vi "ActiView806-Lores.vi"() -> ()   [LabVIEW 2020]
doc: "ActiView is based on a state machine (case structure inside while-loop) with six (orange) states:\n\nState 0: Wait for START, and read/write CFG files\nState 1: Start acquisition, determine speedmode and AD-box version, set panel controls accordingly, stop acquisition\nState 2: Reset panel indicators\nState 3: Initialize saving to BDF file\nState 4: Start acquisition, iterate while-loop to write data to screen and BDF flle (if selected) until STOP is pressed, or error occurs, stop acquisition\nState 5: Reset panel indicators, close BDF file\n\nThe while-loop in (orange) state 4 has five (green) cases.\n\nCase 0: Wait for new data\nCase 1: Read new data from ringbuffer, downsample data, write data to charts and in file array\nCase 2: Transfer block of 1 second of data from file array to BDF file\nCase 3: Close BDF file, and open new BDF file\nCase 4: Calculate average result, and write to ERP graphs \n\nAlso see the Light version of ActiView avalable from the www.biosemi.com"
uses:
  <vilib>/Utility/error.llb/DialogType.ctl
  <vilib>/Utility/config.llb/Read Key (String).vi
  <vilib>/Utility/config.llb/Write Key (String).vi
  <vilib>/Utility/cursorutil.llb/Set Cursor (Icon Pict).vi
  ActiView8-Subvi.llb/StopJazzIni.glb
  ActiView8-Subvi.llb/JazzLoBatWarning.glb
  ActiView8-Subvi.llb/LoBatWarning.glb
  ActiView8-Subvi.llb/StopThreads.glb
  ActiView8-Subvi.llb/TCPidentification.glb
  <vilib>/Utility/inputDevices.llb/keyboardAcquire.vi
  <vilib>/Utility/inputDevices.llb/closeKeyboard.vi
  Instance          61 25Saved   ActiView606-Lores .vi
  <vilib>/Utility/config.llb/NI_LVConfig.lvlib
panel:
  in  "TrigCode":i8(ring) caption="Trigger Format" items=["Analog", "Decimal", "Hexa", "Binary", "Custom"]
  out "Trigger Bar":enum32{"Blank"}(tab)
  out "Dummy String":string
  out "Trigger Chart":i32[][](graph)
  out "Trigger Code":picture
  out "Errors:":i16
  in  "Box":i32(ring) items=["AD-Box 1", "AD-Box 2", "AD-Box 3", "AD-Box 4"]
  out "Right Sidebar":enum32{"Blank"}(tab)
  out "Write":bool
  out "Free on Disk sec":i64=-1 caption="Free on Disc sec"
  out "Nr of Files":i32
  out "Total Saved sec":i32
  out "Current File MB":dbl format="%.1f"
  out "with Jazz":bool
  out "Box4":bool caption="Box1"
  out "Box3":bool caption="Box1"
  out "Box2":bool caption="Box1"
  out "Box1":bool
  in  "FileAppend":bool=TRUE
  in  "RecTimeLimit":i32=9999999 caption="Time Limit (sec)" min=1 max=9999999 step=1
  out "Nr Chan Saved":string="0 + 0"
  out "with AIB":bool
  out "with Sens":bool
  out "with  8 EX":bool
  out "Bandwidth (3dB)":dbl
  in  "Decimation":i8(ring) items=["1", "1/2", "1/4", "1/8", "1/16", "1/32", "1/64"]
  out "Sample Rate":dbl
  in  "FileLimit":i64=999999 caption="File Limit (MB)" min=1 max=999999 step=1
  out "Filepath":string
  out "Save Subset":string
  out "Battery":u8(slide) scale=0.0..100.0
  in  "Marker F8":bool
  in  "Marker F7":bool
  in  "Marker F6":bool
  in  "Marker F5":bool
  in  "Marker F4":bool
  in  "Marker F3":bool
  in  "Marker F2":bool
  in  "Marker F1":bool
  in  "Master Filter Reset":bool
  in  "ScreenLength":i32(ring)=3 caption="Screen Length" items=["1 sec", "2 sec", "4 sec", "8 sec", "16 sec", "32 sec", "64 sec"]
  in  "Start Saving":bool
  in  "Pause Saving":bool
  out "Left Sidebar":T1(tab)
  in  "MonFree":i32[](listbox)=[0, 1, 2, 3, 4, 5, 6, 7, 8, 9, 10, 11, 12, 13, 14, 15, 16, 17, 18, 19, 20, 21, 22, 23, 24, 25, 26, 27, 28, 29, 30, 31, 32, 33, 34, 35, 36, 37, 38, 39, 40, 41, 42, 43, 44, 45, 46, 47, 48, 49, 50, 51, 52, 53, 54, 55, 56, 57, 58, 59, 60, 61, 62, 63, 64, 65, 66, 67, 68, 69, 70, 71, 72, 73, 74, 75, 76, 77, 78, 79, 80, 81, 82, 83, 84, 85, 86, 87, 88, 89, 90, 91, 92, 93, 94, 95, 96, 97, 98, 99, 100, 101, 102, 103, 104, 105, 106, 107, 108, 109, 110, 111, 112, 113, 114, 115, 116, 117, 118, 119, 120, 121, 122, 123, 124, 125, 126, 127, 128, 129, 130, 131, 132, 133, 134, 135, 136, 137, 138, 139, 140, 141, 142, 143, 144, 145, 146, 147, 148, 149, 150, 151, 152, 153, 154, 155, 156, 157, 158, 159, 160, 161, 162, 163, 164, 165, 166, 167, 168, 169, 170, 171, 172, 173, 174, 175, 176, 177, 178, 179, 180, 181, 182, 183, 184, 185, 186, 187, 188, 189, 190, 191, 192, 193, 194, 195, 196, 197, 198, 199, 200, 201, 202, 203, 204, 205, 206, 207, 208, 209, 210, 211, 212, 213, 214, 215, 216, 217, 218, 219, 220, 221, 222, 223, 224, 225, 226, 227, 228, 229, 230, 231, 232, 233, 234, 235, 236, 237, 238, 239, 240, 241, 242, 243, 244, 245, 246, 247, 248, 249, 250, 251, 252, 253, 254, 255]
  in  "Reference":i8(ring) items=["None (raw)", "Avg of 264", "Avg 1-256", "Avg 1-160", "Avg 1-128", "Avg 1-64", "Avg 1-32", "Avg of Displ", "Free Choice"]
  in  "Mon Filter Reset":bool
  in  "MonLP":bool=TRUE caption="Lowpass"
  in  "MonHP":bool=TRUE caption="Highpass"
  in  "RefFree":i32[](listbox)
  in  "Channels":i8(ring) items=["All 264 Chan ", "A-H (256)", "A-E (160)", "ABCD (128)", "A+B (64)", "A (32)", "B (32)", "C (32)", "D (32)", "E (32)", "F (32)", "G (32)", "H(32)", "EXG (8)", "Free Choice"]
  in  "MonHPfreq":dbl=0.16 caption="Cutoff Freq" min=0.01 max=9.99 step=0.1 format="%.2f"
  in  "MonScale":i8(ring)=4 caption="Y-scale\nVolts/div" items=["5 uV", "10 uV", "20 uV", "50 uV", "100 uV", "200 uV", "500 uV", "1 mV", "2 mV", "5 mV", "10 mV", "20 mV", "50 mV", "100 mV", "200 mV", "500 mV"]
  in  "MonLPfreq":dbl=100.0 caption="Cutoff Freq" min=1.0 max=8191.0 step=10.0
  out "NoRef Blinker":bool
  in  "AddTP":bool caption="Add  8 EXG"
  in  "BipFree":i32[](listbox)=[0, 2, 4, 6] caption="Bipolar\nLeads"
  in  "Bip Filter Reset":bool
  in  "BipLP":bool=TRUE caption="Lowpass"
  in  "BipHP":bool=TRUE caption="Highpass"
  in  "BipHPfreq":dbl=0.16 caption="Cutoff Freq" min=0.01 max=99.9 step=1.0 format="%.2f"
  in  "BipScale":i8(ring)=7 caption="Y-scale\nVolts/div" items=["5 uV", "10 uV", "20 uV", "50 uV", "100 uV", "200 uV", "500 uV", "1 mV", "2 mV", "5 mV", "10 mV", "20 mV", "50 mV", "100 mV", "200 mV", "500 mV"]
  in  "BipLPfreq":dbl=100.0 caption="Cutoff Freq" min=1.0 max=8191.0 step=10.0
  out "TP Offset Graph 2":dbl[](graph) caption="EX5 - EX8"
  out "TP Offset Graph 1":dbl[](graph) caption="EX1 - EX4"
  in  "Offset":i8(ring) caption="Channel\nSelection" items=["All 256 Chan ", "A + B", "C + D", "E + F", "G + H"]
  out "Full Range":bool=TRUE
  in  "OffsetScale":i8(ring)=3 caption="Displayed \nRange" items=["20 mV", "50 mV", "100 mV", "262  mV", "1049 mV"]
  out "Rejected Sweeps":i32
  out "Valid Sweeps":i32
  in  "AvgLP":bool caption="Lowpass"
  in  "AvgLPfreq":dbl=100.0 caption="Cuttoff Freq" min=1.0 max=8191.0 step=10.0
  in  "AvgTrigLog":i8(ring) items=["AND trigs ", "OR trigs"]
  in  "AvgTrigSel":i32[](listbox)=[0]
  in  "AvgHP":bool=TRUE caption="Highpass"
  in  "AvgHPfreq":dbl=1.0 caption="Cutoff Freq" min=0.1 max=99.9 step=10.0 format="%.1f"
  out "RejDif":bool caption="Reject"
  out "RejAbs":bool caption="Reject"
  in  "AvgRelReject":dbl=50.0 caption="Difference with\navg more than:" min=0.0 step=1.0 format="%.1f"
  in  "AvgAbsReject":dbl=200.0 caption="All  sweeps\nlarger than:" min=0.0 step=10.0
  in  "AvgSweep":i32=500 caption="Sweep Length" min=1 max=9999 step=100
  in  "AvgAutoscale":bool=TRUE caption="Autoscale"
  in  "AvgScale":dbl=5.0 caption="Y-scale in uV" min=0.0 format="%.1f"
  in  "Averaging":bool
  out "Battery\nCapacitance":u8(slide) caption="Battery" scale=0.0..100.0
  in  "Aux DC Reset":bool
  in  "AuxReset":bool=TRUE caption="Reset at \nScreen Start"
  out "GSR units":string="?"
  out "GSR2":dbl format="%_3f"
  out "GSR1":dbl format="%_3f"
  out "GSR2 pos":bool
  out "GSR2 neg":bool
  out "GSR1 pos":bool
  in  "GsrScale":i8(ring)=4 caption="GSR Y-scale" items=["1", "2", "5", "10", "20", "50", "100", "200", "500", "1k", "2k", "5k", "10k", "20k", "50k", "100k", "200k", "500k", "1M"]
  out "GSR1 neg":bool
  in  "ErgoLP":bool caption="Lowpass"
  in  "ErgoScale":i8(ring)=6 caption="Ergo Y-Scale" items=["5 uV", "10 uV", "20 uV", "50 uV", "100 uV", "200 uV", "500 uV", "1 mV", "2 mV", "5 mV", "10 mV", "20 mV", "50 mV", "100 mV", "200 mV", "500 mV", "1V", "2V", "4V"]
  in  "AuxFree":i32[](listbox)=[0, 1, 2, 3, 4, 5, 6] caption="Sensors"
  out "Degrees Celcius":dbl format="%.2f"
  in  "TempScale":i8(ring)=3 caption="Temp Y-scale" items=["0.01 C", "0.02 C", "0.05  C", "0.1 C", "0.2 C", "0.5 C", "1 C", "2 C", "5  C", "10 C"]
  in  "PletScale":i8(ring)=7 caption="Plet Y-scale" items=["5 uV", "10 uV", "20 uV", "50 uV", "100 uV", "200 uV", "500 uV", "1 mV", "2 mV", "5 mV", "10 mV", "20 mV", "50 mV", "100 mV", "200 mV", "500 mV"]
  in  "RespScale":i8(ring)=4 caption="Resp Y-scale" items=["0.1 mV", "0.2 mV", "0.5  mV", "1 mV", "2 mV", "5 mV", "10 mV", "20 mV", "50 mV", "100 mV", "200 mV", "500 mV"]
  in  "JazzOn":bool caption="Enable Jazz"
  in  "JazzReset":bool=TRUE caption="DC Reset at\nScreen Start"
  in  "Jazz Filter Reset":bool
  in  "JazzFree":i32[](listbox)=[0, 1, 2, 3, 4, 5, 6, 7] caption="Jazz\nChannels"
  out "Jazz Batt Perc":string
  out "Jazz Batt Cap":u8(slide) caption="Jazz Batt" scale=0.0..100.0
  out "Jazz New\nFirmware":bool
  in  "AnaFree":i32[](listbox)=[0, 1, 2, 3, 4, 5, 6, 7, 8, 9, 10, 11, 12, 13, 14, 15] caption="AIB\nChannels"
  in  "AnaReset":bool=TRUE caption="Reset at \nScreen Start"
  out "Ana Offset Graph":dbl[](graph)
  in  "AnaOffset":i32(ring) caption="AIB Channel" items=["Ana1", "Ana2", "Ana3", "Ana4", "Ana5", "Ana6", "Ana7", "Ana8", "Ana9", "Ana10", "Ana11", "Ana12", "Ana13", "Ana14", "Ana15", "Ana16", "Ana17", "Ana18", "Ana19", "Ana20", "Ana21", "Ana22", "Ana23", "Ana24", "Ana25", "Ana26", "Ana27", "Ana28", "Ana29", "Ana30", "Ana31", "Ana32"]
  in  "Ana Filter Reset":bool
  in  "AnaLP":bool=TRUE caption="Lowpass"
  in  "AnaHP":bool=TRUE caption="Highpass"
  in  "AnaHPfreq":dbl=0.16 caption="Cutoff Freq" min=0.01 max=4095.0 step=1.0 format="%.2f"
  in  "AnaScale":i8(ring)=7 caption="Y-scale\nVolts/div" items=["5 uV", "10 uV", "20 uV", "50 uV", "100 uV", "200 uV", "500 uV", "1 mV", "2 mV", "5 mV", "10 mV", "20 mV", "50 mV", "100 mV", "200 mV", "500 mV", "1 V", "2 V", "4 V"]
  in  "AnaLPfreq":dbl=100.0 caption="Cutoff Freq" min=1.0 max=8191.0 step=10.0
  in  "Buffer":i8(ring)=2 caption="Ringbuffer Size" items=["8 Mbyte", "16 Mbyte", "32 Mbyte", "64 Mbyte"]
  out "Pause Off/On":string="-1 / -1"
  out "Write CFG":bool
  in  "Save Configuration File":bool
  out "Current Filepath":string
  in  "Load Configuration File":bool
  in  "Start":bool
  out "Low Battery":bool
  out "CM in Range":bool
  out "Ring Buffer":cluster{dbl, dbl}(knob)={0.0033134730043177896, 0.0033134730043177896} scale=0.0..32.0
  in  "Stop":bool
  in  "Charts/Graphs":T2(tab)
  out "Mon Chart":dbl[][](graph)
  out "Trace61":string
  out "Trace60":string
  out "Trace59":string
  out "Trace58":string
  out "Trace57":string
  out "Trace56":string
  out "Trace55":string
  out "Trace54":string
  out "Trace53":string
  out "Trace52":string
  out "Trace51":string
  out "Trace50":string
  out "Trace49":string
  out "Trace48":string
  out "Trace47":string
  out "Trace46":string
  out "Trace45":string
  out "Trace44":string
  out "Trace43":string
  out "Trace42":string
  out "Trace41":string
  out "Trace40":string
  out "Trace39":string
  out "Trace38":string
  out "Trace37":string
  out "Trace36":string
  out "Trace35":string
  out "Trace34":string
  out "Trace33":string
  out "Trace32":string
  out "Trace31":string
  out "Trace30":string
  out "Trace29":string
  out "Trace28":string
  out "Trace27":string
  out "Trace26":string
  out "Trace25":string
  out "Trace24":string
  out "Trace23":string
  out "Trace22":string
  out "Trace21":string
  out "Trace20":string
  out "Trace19":string
  out "Trace18":string
  out "Trace17":string
  out "Trace16":string
  out "Trace15":string
  out "Trace14":string
  out "Trace13":string
  out "Trace12":string
  out "Trace10":string
  out "Trace9":string
  out "Trace8":string
  out "Trace7":string
  out "Trace6":string
  out "Trace5":string
  out "Trace4":string
  out "Trace3":string
  out "Trace2":string
  out "Trace1":string
  out "Trace64":string
  out "Trace63":string
  out "Trace62":string
  out "Trace11":string
  out "Bip8":string
  out "Bip7":string
  out "Bip6":string
  out "Bip5":string
  out "Bip4":string
  out "Bip3":string
  out "Bip2":string
  out "Bip1":string
  out "Bip Chart":dbl[][](graph)
  out "Offset33":string
  out "Offset64":string
  out "Offset63":string
  out "Offset62":string
  out "Offset61":string
  out "Offset60":string
  out "Offset59":string
  out "Offset58":string
  out "Offset57":string
  out "Offset56":string
  out "Offset55":string
  out "Offset54":string
  out "Offset53":string
  out "Offset52":string
  out "Offset51":string
  out "Offset50":string
  out "Offset49":string
  out "Offset Graph First Half":dbl[](graph)
  out "Offset48":string
  out "Offset47":string
  out "Offset46":string
  out "Offset45":string
  out "Offset44":string
  out "Offset43":string
  out "Offset42":string
  out "Offset41":string
  out "Offset40":string
  out "Offset39":string
  out "Offset38":string
  out "Offset37":string
  out "Offset36":string
  out "Offset35":string
  out "Offset34":string
  out "Offset32":string
  out "Offset31":string
  out "Offset30":string
  out "Offset29":string
  out "Offset28":string
  out "Offset27":string
  out "Offset26":string
  out "Offset25":string
  out "Offset24":string
  out "Offset23":string
  out "Offset22":string
  out "Offset21":string
  out "Offset20":string
  out "Offset19":string
  out "Offset18":string
  out "Offset17":string
  out "Offset16":string
  out "Offset15":string
  out "Offset14":string
  out "Offset13":string
  out "Offset12":string
  out "Offset11":string
  out "Offset10":string
  out "Offset9":string
  out "Offset8":string
  out "Offset7":string
  out "Offset6":string
  out "Offset5":string
  out "Offset4":string
  out "Offset3":string
  out "Offset2":string
  out "Offset1":string
  out "Offset Graph  Second Half":dbl[](graph)
  out "Avg2":dbl[][](graph) caption="Avg 2"
  out "Avg1":dbl[][](graph) caption="Avg 1"
  in  "RefFreeAvg2":i32[](listbox)
  in  "MonFreeAvg2":i32(listbox)=1
  in  "RefFreeAvg1":i32[](listbox)
  in  "MonFreeAvg1":i32(listbox)
  out "Sweeping":bool
  out "Aux7":string
  out "Aux6":string
  out "Aux5":string
  out "Aux4":string
  out "Aux Chart":dbl[][](graph)
  out "Aux3":string
  out "Aux2":string
  out "Aux1":string
  out "Jazz9":string
  out "Jazz8":string
  out "Jazz7":string
  out "Jazz6":string
  out "Jazz5":string
  out "Jazz4":string
  out "Jazz Chart":dbl[][](graph)
  out "Jazz3":string
  out "Jazz2":string
  out "Jazz1":string
  out "Ana17":string
  out "Ana18":string
  out "Ana19":string
  out "Ana20":string
  out "Ana21":string
  out "Ana32":string
  out "Ana31":string
  out "Ana30":string
  out "Ana29":string
  out "Ana28":string
  out "Ana27":string
  out "Ana26":string
  out "Ana25":string
  out "Ana22":string
  out "Ana23":string
  out "Ana24":string
  out "Ana Chart":dbl[][](graph)
  out "Ana1":string
  out "Ana2":string
  out "Ana3":string
  out "Ana4":string
  out "Ana5":string
  out "Ana16":string
  out "Ana15":string
  out "Ana14":string
  out "Ana13":string
  out "Ana12":string
  out "Ana11":string
  out "Ana10":string
  out "Ana9":string
  out "Ana6":string
  out "Ana7":string
  out "Ana8":string
  in  "TCPaddJazz":bool caption="Add 9 Jazz"
  in  "TCPaddTrig":bool caption="Add Trigger/Status Chan"
  out "Bytes in TCP Array":i32
  out "Bytes received by Client":i32
  out "TCP samples/channel":i32
  out "Channels sent by TCP":i32
  in  "TCPaddAnas":bool caption="Add 32 AIB Chan"
  in  "TCPaddSens":bool caption="Add 7 Sensors"
  in  "TCPaddTP":bool caption="Add  8 EX  electrodes"
  in  "TCPsubset":i8(ring)=7 caption="TCP subset:" items=["A1 - H32 (256)", "A1 - E32 (160)", "A1 - D32 (128)", "A1 - B32 (64)", "A1 - A32 (32)", "A1 - A16 (16)", "A1 -A8 (8)", "None (0) "]
  out "TCP Listening":bool
  out "TCP Connected":bool
  out "Remote Address":string
  out "Receive Remote Port":u16
  out "Bytes sent by Server":i32
  in  "LocalPort":u16=778 caption="Sent Local Port"
  out "Application:Kind":T3(ring)
  out "AD-box":string="?"
  out "Speed Mode":i8=-1
  in  "Edit":bool
  # "Trig 1 - 8"
  # "Trig 9-16"
  # "BDF File"
  # "Hz"
  # "Hz"
  # "AD-Box"
  # "Hz"
  # "Hz"
  # "None = CMS"
  # "Hz"
  # "Hz"
  # "ms"
  # "Hz"
  # "Hz"
  # "uV"
  # "uV"
  # "uV"
  # "GSR\nIn Range"
  # "1"
  # "2"
  # "C"
  # "Hz"
  # "Hz"
  # "Range in mV"
  # "Versus"
  # "Versus"
  # "ActiView"
  # "data-acquisition software for ActiveTwo measurement system"
  # "Version 8.0, February 13, 2018"
  # "Push to edit source code (LabVIEW licensees only)"
  # "www.biosemi.com\nmetting@biosemi.com\n+31 20 3302956\n+31 650 626354 (emergencies)"
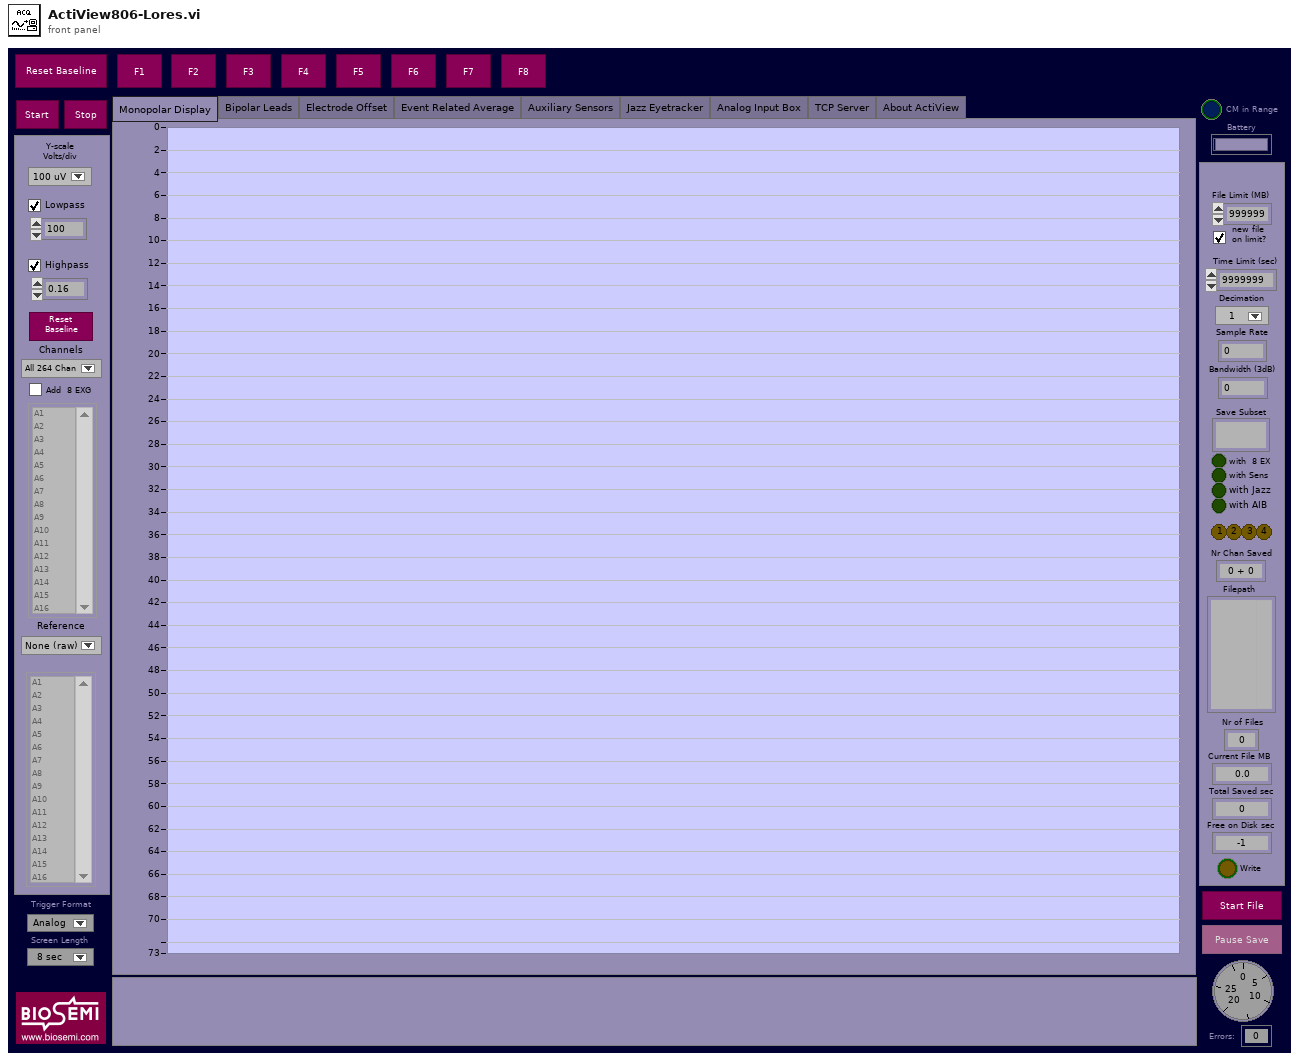
[diagram p1: front panel]
types:
  T1 = enum32{"Monopolar", "Bipolar", "Offset", "Average", "Sensors", "Jazz", "Analog", "Initialization"}
  T2 = enum32{"Monopolar Display", "Bipolar Leads", "Electrode Offset", "Event Related Average", "Auxiliary Sensors", "Jazz Eyetracker", "Analog Input Box", "TCP Server", "About ActiView"}
  T3 = enum32{"invalid app kind", "Development System", "Run Time System", "Student Edition", "Embedded LabVIEW", "Evaluation", "Custom"}
  T4 = enum32{"Page Enabled", "Page Disabled", "Page Disabled & Grayed"}
  T5 = enum8{"Enabled", "Disabled", "Disabled and Grayed Out"}
  T6 = cluster{"Warning":i8, "Motherboard":i8, "ElecGain":i8, "RespSwitch":i8, "LineWidth":u8, "Cursor":u16, "PopupKiller":i8, "BreathBelt":i8}
  T7 = cluster{"Mark2":bool, "GSR16Hz":bool, "JazzRec":bool, "Speed Mode":i8, "ADC Rate":i32, "ADC Channels":i32, "Screen Ratio":i32, "Decimate Ratio":i32, "Mon Channels":i32, "Bip Channels":i32, "Aux Channels":i32, "Jazz Channels":i32, "Ana Channels":i32, "Save Subset":i8, "Add Touchproofs":bool, "Add Sensors":bool, "Add Jazz":bool, "Add Anas":bool, "Save Box":u32, "PauseOff":i32, "PauseOn":i32, "Save Path":path}
  T8 = cluster{"All Labels":string[], "Spec Labels":string[]}
  T9 = cluster{"connection ID":refnum<k5>, "remote address":string, "remote port":u16}
  T10 = enum16{"open", "replace", "create", "open or create", "replace or create", "replace or create with confirmation"}
  T11 = cluster{"Start Averaging":bool, "Busy Averaging":bool, "Sweep Lenght in Samples":i32, "Valid Sweeps":i32, "Rejected Sweeps":i32, "First Graph Update":bool}
  T12 = enum16{"0", "1", "2", "3", "4", "5", "6", "7", "8", "9", "A", "B", "C", "D", "E", "F", "G", "H", "I", "J", "K", "L", "M", "N", "O", "P", "Q", "R", "S", "T", "U", "V", "W", "X", "Y", "Z", "F1", "F2", "F3", "F4", "F5", "F6", "F7", "F8", "F9", "F10", "F11", "F12", "F13", "F14", "F15", "ADD", "BACK", "BACKSLASH", "CAPITAL", "COMMA", "DECIMAL", "DELETE", "DIVIDE", "DOWN", "END", "EQUALS", "ESCAPE", "GRAVE (`)", "HOME", "INSERT", "LBRACKET", "LCONTROL", "LEFT", "L ALT", "LSHIFT", "LWIN", "MINUS", "MULTIPLY", "NEXT", "NUMLOCK", "NUMPAD_0", "NUMPAD_1", "NUMPAD_2", "NUMPAD_3", "NUMPAD_4", "NUMPAD_5", "NUMPAD_6", "NUMPAD_7", "NUMPAD_8", "NUMPAD_9", "PAUSE", "PERIOD", "PRIOR (PG UP)", "RBRACKET", "RCONTROL", "RETURN", "RIGHT", "R ALT", "RSHIFT", "RWIN", "SCROLL", "SEMICOLON", "SLASH", "SPACE", "SUBTRACT", "TAB", "UP", "ENTER (num pad)", "' (quote)"}
  T13 = cluster{"Font Name:":string, "Size":i16, "Strikeout?":bool, "Italic?":bool, "Underline?":bool, "Outline?":bool, "Shadow?":bool, "Bold?":bool}
  T14 = cluster{"Jazz No Data":bool, "Jazz Packet Loss":bool, "Jazz Batt":u8, "Jazz Packet Loss 2":bool}
  T15 = cluster{"GSR2pos":bool, "GSR1neg":bool, "GSR1pos":bool, "GSR2neg":bool}
  T16 = cluster{"Sweeping":bool, "RejAbs":bool, "RejDif":bool}
  T17 = cluster{"Speed Mode":i8, "Save Subset":i8, "Initially Channel Selection":i32[], "Add Touchproofs":bool, "Mon Channels":i32, "Bip Channels":i32, "Add Sensors":bool, "Initially Channel Selection":i32[], "Add Jazz":bool, "Initially Channel Selection":i32[], "Add Anas":bool, "Initially Channel Selection":i32[], "Save Box":u32}
  T18 = typedef "DialogType.ctl" = u16
  T19 = typedef "NI_LVConfig.lvlib/Config Data RefNum.ctl" = refnum<k1>
  T20 = cluster{"Save Subset":i8, "Add Touchproofs":bool, "Add Sensors":bool, "Add Jazz":bool, "Add Anas":bool, "Save Box":u32}
  T21 = cluster{"Local Patient Identification":string, "Local  Recording Identification":string}
  T22 = cluster{"Mark2":bool, "GSR16Hz":bool, bool, "Speed Mode":i8}
  T23 = typedef "AVTCP-TCP Options.ctl" = cluster{"Subset":i32, "EX":bool}
  T24 = cluster{"length":i32, "f":i32, "f":i32, "f":i32, "f":i32, "f":i32}
  T25 = cluster{bool, bool, bool, bool, bool, bool, bool, bool}
  T26 = cluster{"Clear Block":i32, "Screen Ratio":dbl, "Y1":i16, "Y2":i16, "Y3":i16, "Color":u32}
  T27 = cluster{"Sync Errors":i16, "Recent Sync Error":bool}
  T28 = cluster{"LoBatChange":bool, "JazzLoBatChange":bool}
  T29 = enum16{"0", "1", "2", "3", "4", "5", "6", "7", "8", "9", "A", "B", "C", "D", "E", "F", "G", "H", "I", "J", "K", "L", "M", "N", "O", "P", "Q", "R", "S", "T", "U", "V", "W", "X", "Y", "Z", "F1", "F2", "F3", "F4", "F5", "F6", "F7", "F8", "F9", "F10", "F11", "F12", "F13", "F14", "F15", "ADD", "BACK", "BACKSLASH", "CAPITAL", "COMMA", "DECIMAL", "DELETE", "DIVIDE", "DOWN", "END", "EQUALS", "ESCAPE", "GRAVE (`)", "HOME", "INSERT", "LBRACKET", "LCONTROL", "LEFT", "L ALT", "LSHIFT", "LWIN", "MINUS", "MULTIPLY", "NEXT", "NUMLOCK", "NUMPAD_0", "NUMPAD_1", "NUMPAD_2", "NUMPAD_3", "NUMPAD_4", "NUMPAD_5", "NUMPAD_6", "NUMPAD_7", "NUMPAD_8", "NUMPAD_9", "PAUSE", "PERIOD", "PRIOR (PG UP)", "RBRACKET", "RCONTROL", "RETURN", "RIGHT", "R ALT", "RSHIFT", "RWIN", "SCROLL", "SEMICOLON", "SLASH", "SPACE", "SUBTRACT", "TAB", "UP", "ENTER (num pad)", "' (quote)"}[]
  T30 = cluster{"GsrScale":i8, "ErgoScale":i8, "ErgoLP":bool, "RespScale":i8, "PletScale":i8, "TempScale":i8}
  T31 = cluster{"Mon Channels":i32, "Bip Channels":i32, "Aux Channels":i32, "Jazz Channels":i32}
  T32 = cluster{"End of Screen":bool, "Prop Screen Minimum":i64, "Screen Position":i32}
  T33 = cluster{"Ring Buffer Overflow":bool, "First Call":bool}
  T34 = cluster{"GSR1pos":bool, "GSR1neg":bool, "GSR2pos":bool, "GSR2neg":bool}
  T35 = cluster{"Jazz No Data":bool, "Jazz Packet Loss":bool, "Jazz Batt":u8, "Jazz New Firmware":bool}
  T36 = cluster{"Xo":dbl, "Xmax":dbl, "Xmin":dbl, "Marker values":dbl[]}
  T37 = cluster{"AvgLP":bool, "AvgLPfreq ":dbl, "AvgHP":bool, "AvgHPfreq":dbl}
  T38 = cluster{"MonLP":bool, "MonLPfreq":dbl, "MonHP":bool, "MonHPfreq":dbl}
  T39 = cluster{"BipLP":bool, "BipLPfreq":dbl, "BipHP":bool, "BipHPfreq":dbl}
  T40 = cluster{"AnaLP":bool, "AnaLPfreq":dbl, "AnaHP":bool, "AnaHPfreq":dbl}
  T41 = cluster{"Speed Mode":i8, "Save Subset":i8, i32[], "Add Touchproofs":bool, "Mon Channels":i32, "Bip Channels":i32, "Add Sensors":bool, i32[], "Add Jazz":bool, i32[], "Add Anas":bool, i32[], "Save Box":u32}
  T42 = cluster{"Marker F1":bool, "Marker F2":bool, "Marker F3":bool, "Marker F4":bool, "Marker F5":bool, "Marker F6":bool, "Marker F7":bool, "Marker F8":bool}
diagram:
  w2 = i8 0  # BreathBelt
  w4 = FALSE  # JazzRec
  w7 = FALSE  # Add Anas
  w9 = 0  # Ana Channels
  w5 = FALSE  # GSR16Hz
  w14 = u32 0  # Save Box
  w6 = FALSE  # Mark2
  w17 = path ""  # Save Path
  w15 = 0  # PauseOff
  w16 = 0  # PauseOn
  w19 = 0  # ADC Rate
  w20 = 0  # ADC Channels
  w22 = 0  # Screen Ratio
  w8 = FALSE  # Add Jazz
  w10 = 0  # Jazz Channels
  w11 = FALSE  # Add Sensors
  w12 = FALSE  # Add Touchproofs
  w13 = i8 0  # Save Subset
  w18 = i8 -1  # Speed Mode
  w21 = 0  # Aux Channels
  w24 = 0  # Bip Channels
  w23 = 0  # Decimate Ratio
  w25 = 0  # Mon Channels
  w26 = i8 0  # PopupKiller
  w31 = FALSE  # Initially Not Start with Save
  w34 = refnum<file> refnum  # Dummy Refnum
  w27 = u16 0  # Cursor
  w28 = u8 0  # LineWidth
  w29 = i8 -1  # RespSwitch
  w37 = i8 -1  # Warning
  w39 = i8 -1  # Motherboard
  w38 = i8 -1  # ElecGain
  w40 = FALSE  # Initially Not Config Changed
  w42 = string[] []  # Spec Labels
  w43 = string[] []  # All Labels
  w30 = i32[] []  # Initially Channel Selection
  w32 = 0  # Initially  nothing saved
  w45 = FALSE  # Initially Not Busy Saving
  w44 = 0  # Initial State
  n1 = stacked-sequence {
    tunnel: [w74] -> w35
    frame #0 {
      w46 = T5."Enabled" ("Disabled")
      w47 = 0.5 ("X Scale.Range:Minimum")
      w48 = 128.5 ("X Scale.Range:Maximum")
      w51 = 8191.0 ("Data Range:Maximum")
      w74 = errorcluster {"status"=FALSE, "code"=0, "source"=""}  # Initially  No Error
      w75 = i32[] [] ("Disabled Items []")
      w72 = FALSE ("Visible")
      n2 = for {
        N: 264 -> [_]
        tunnel: [w90] -> w76 mode=indexing
        i -> [w95]
        n3 = Quotient & Remainder(x=w95, y=32) -> (x-y*floor(x/y)=w92:i32, floor(x/y)=w93:i32)
        n4 = case shown="8" w93 {
          tunnel: ["A" "B" "C" "D" "E" "F" "G" "H" "EX"] -> w91
          frame 0, Default {
          }
          frame 1 {
          }
          frame 2 {
          }
          frame 3 {
          }
          frame 4 {
          }
          frame 5 {
          }
          frame 6 {
          }
          frame 7 {
          }
          frame 8 {
          }
        }
        n5 = Increment(x=w92) -> (x+1=w89:i32)
        n6 = Format Into String(initial string=w91, w89) -> (resulting string=w90:string)  [unwired: 2 in, 1 out]
      }
      n7 = for {
        N: 128 -> [_]
        tunnel: [w79] -> w49 mode=indexing
        i -> [w81]
        n8 = Increment(x=w81) -> (x+1=w80:i32)
        n9 = To Double Precision Float(number=w80) -> (double precision float=w79:dbl)
      }
      n10 = Increment(x=264) -> (x+1=w56:i32)
      n11 = Increment(x=8) -> (x+1=w55:i32)
      n12 = Increment(x=7) -> (x+1=w54:i32)
      n13 = Increment(x=9) -> (x+1=w53:i32)
      n14 = Increment(x=32) -> (x+1=w52:i32)
      n15 = property on="Charts/Graphs" class="TabCtl (strict)"() -> ("Pages"=w73:refnum<vi>[])  [unwired: 2 in, 2 out]
      n16 = property on="Low Battery" class="Bool (strict)"("Visible"=w72) -> ()  [unwired: 2 in, 2 out]
      n17 = for {
        N: w54 -> [_]
        tunnel: [w84] -> w64 mode=indexing
        i -> [w84]
      }
      n18 = for {
        N: w53 -> [_]
        tunnel: [w83] -> w61 mode=indexing
        i -> [w83]
      }
      n19 = property on="NoRef Blinker" class="Bool"("Visible"=w72) -> ()  [unwired: 2 in, 2 out]
      n20 = property on="Box" class="Ring (strict)"("Visible"=w72) -> ()  [unwired: 2 in, 2 out]
      n21 = for {
        N: w55 -> [_]
        tunnel: [w85] -> w67 mode=indexing
        i -> [w85]
      }
      n22 = for {
        N: w52 -> [_]
        tunnel: [w82] -> w58 mode=indexing
        i -> [w82]
      }
      n23 = for {
        N: w56 -> [_]
        tunnel: [w86] -> w70 mode=indexing
        i -> [w86]
      }
      n24 = for {
        tunnel: w73 -> [w88] mode=indexing
        n25 = property class="Page"(reference=w88, "Page Enabled State"=T4."Page Enabled") -> ()  [unwired: 1 in, 2 out]
      }
      n26 = property on="AddTP" class="Bool (strict)"("Disabled"=w46) -> ()  [unwired: 2 in, 2 out]
      n27 = property on="TP Offset Graph 1" class="WFGraph (strict)"("Disabled"=w46) -> ()  [unwired: 2 in, 2 out]
      n28 = property on="TP Offset Graph 2" class="WFGraph (strict)"("Disabled"=w46) -> ()  [unwired: 2 in, 2 out]
      n29 = property on="GSR1 pos" class="Bool (strict)"("Disabled"=w46) -> ()  [unwired: 2 in, 2 out]
      n30 = property on="GSR1 neg" class="Bool (strict)"("Disabled"=w46) -> ()  [unwired: 2 in, 2 out]
      n31 = property on="GSR1" class="DigNum (strict)"("Disabled"=w46) -> ()  [unwired: 2 in, 2 out]
      n32 = property on="GSR2 neg" class="Bool (strict)"("Disabled"=w46) -> ()  [unwired: 2 in, 2 out]
      n33 = property on="GSR2 pos" class="Bool (strict)"("Disabled"=w46) -> ()  [unwired: 2 in, 2 out]
      n34 = property on="GsrScale" class="Ring (strict)"("Disabled"=w46) -> ()  [unwired: 2 in, 2 out]
      n35 = property on="GSR units" class="Str"("Disabled"=w46) -> ()  [unwired: 2 in, 2 out]
      n36 = property on="ErgoScale" class="Ring (strict)"("Disabled"=w46) -> ()  [unwired: 2 in, 2 out]
      n37 = property on="ErgoLP" class="Bool (strict)"("Disabled"=w46) -> ()  [unwired: 2 in, 2 out]
      n38 = property on="RespScale" class="Ring (strict)"("Disabled"=w46) -> ()  [unwired: 2 in, 2 out]
      n39 = property on="PletScale" class="Ring (strict)"("Disabled"=w46) -> ()  [unwired: 2 in, 2 out]
      n40 = property on="TempScale" class="Ring (strict)"("Disabled"=w46) -> ()  [unwired: 2 in, 2 out]
      n41 = property on="Degrees Celcius" class="DigNum (strict)"("Disabled"=w46) -> ()  [unwired: 2 in, 2 out]
      n42 = property on="JazzOn" class="Bool (strict)"("Disabled"=w46) -> ()  [unwired: 2 in, 2 out]
      n43 = To Double Precision Float(number=w70) -> (double precision float=w69:dbl[])
      n44 = To Double Precision Float(number=w67) -> (double precision float=w66:dbl[])
      n45 = To Double Precision Float(number=w64) -> (double precision float=w63:dbl[])
      n46 = To Double Precision Float(number=w61) -> (double precision float=w60:dbl[])
      n47 = To Double Precision Float(number=w58) -> (double precision float=w57:dbl[])
      n48 = property on="ScreenLength" class="Ring (strict)"("Disabled Items []"=w75) -> ()  [unwired: 2 in, 2 out]
      n49 = property on="Channels" class="Ring (strict)"("Disabled Items []"=w75) -> ()  [unwired: 2 in, 2 out]
      n50 = property on="Reference" class="Ring (strict)"("Disabled Items []"=w75) -> ()  [unwired: 2 in, 2 out]
      n51 = property on="Offset" class="Ring (strict)"("Disabled Items []"=w75) -> ()  [unwired: 2 in, 2 out]
      n52 = property on="TCPsubset" class="Ring (strict)"("Disabled Items []"=w75) -> ()  [unwired: 2 in, 2 out]
      n53 = property on="Offset Graph First Half" class="WFGraph (strict)"("XScale.Maximum"=w48, "XScale.Minimum"=w47, "XScale.MarkerVals[]"=w49) -> ()  [unwired: 2 in, 2 out]
      n54 = property on="Offset Graph  Second Half" class="WFGraph (strict)"("XScale.Maximum"=w48, "XScale.Minimum"=w47, "XScale.MarkerVals[]"=w49) -> ()  [unwired: 2 in, 2 out]
      n55 = property on="Mon Chart" class="WFChart (strict)"("YScale.MarkerVals[]"=w69) -> ()  [unwired: 2 in, 2 out]
      n56 = property on="Bip Chart" class="WFChart (strict)"("YScale.MarkerVals[]"=w66) -> ()  [unwired: 2 in, 2 out]
      n57 = property on="Aux Chart" class="WFChart (strict)"("YScale.MarkerVals[]"=w63) -> ()  [unwired: 2 in, 2 out]
      n58 = property on="Jazz Chart" class="WFChart (strict)"("YScale.MarkerVals[]"=w60) -> ()  [unwired: 2 in, 2 out]
      n59 = property on="Ana Chart" class="WFChart (strict)"("YScale.MarkerVals[]"=w57) -> ()  [unwired: 2 in, 2 out]
      n60 = property on="BipLPfreq" class="DigNum (strict)"("Data Range:Maximum"=w51) -> ()  [unwired: 2 in, 2 out]
      n61 = property on="AvgLPfreq" class="DigNum (strict)"("Data Range:Maximum"=w51) -> ()  [unwired: 2 in, 2 out]
      n62 = property on="AnaLPfreq" class="DigNum (strict)"("Data Range:Maximum"=w51) -> ()  [unwired: 2 in, 2 out]
      n63 = property on="MonLPfreq" class="DigNum (strict)"("Data Range:Maximum"=w51) -> ()  [unwired: 2 in, 2 out]
      n64 = property on="MonFree" class="LstBox (strict)"("Item Names"=w76) -> ()  [unwired: 2 in, 2 out]
      n65 = property on="RefFree" class="LstBox (strict)"("Item Names"=w76) -> ()  [unwired: 2 in, 2 out]
      n66 = property on="MonFreeAvg1" class="LstBox (strict)"("Item Names"=w76) -> ()  [unwired: 2 in, 2 out]
      n67 = property on="RefFreeAvg1" class="LstBox (strict)"("Item Names"=w76) -> ()  [unwired: 2 in, 2 out]
      n68 = property on="MonFreeAvg2" class="LstBox (strict)"("Item Names"=w76) -> ()  [unwired: 2 in, 2 out]
      n69 = property on="RefFreeAvg2" class="LstBox (strict)"("Item Names"=w76) -> ()  [unwired: 2 in, 2 out]
      n70 = property on="Battery" class="Slide (strict)"("Visible"=TRUE) -> ()  [unwired: 2 in, 2 out]
    }
  }
  n71 = vi-ref "AVTCP-Server.vi"() -> (w1:refnum<vi>)
  n72 = invoke on="Control server" class="SubPnl" method="Insert VI"("VI Ref"=w1) -> ()  [unwired: 3 in, 4 out]
  n73 = call "AVTCP-Server.vi"() -> ()  [unwired: 12 in]
  n74 = Bundle("Warning"=w37, "Motherboard"=w39, "ElecGain"=w38, "RespSwitch"=w29, "LineWidth"=w28, "Cursor"=w27, "PopupKiller"=w26, "BreathBelt"=w2) -> (w36:T6)  [unwired: 1 out]
  n75 = Bundle("Mark2"=w6, "GSR16Hz"=w5, "JazzRec"=w4, "Speed Mode"=w18, "ADC Rate"=w19, "ADC Channels"=w20, "Screen Ratio"=w22, "Decimate Ratio"=w23, "Mon Channels"=w25, "Bip Channels"=w24, "Aux Channels"=w21, "Jazz Channels"=w10, "Ana Channels"=w9, "Save Subset"=w13, "Add Touchproofs"=w12, "Add Sensors"=w11, "Add Jazz"=w8, "Add Anas"=w7, "Save Box"=w14, "PauseOff"=w15, "PauseOn"=w16, "Save Path"=w17) -> (w3:T7)  [unwired: 1 out]
  n76 = Bundle("All Labels"=w43, "Spec Labels"=w42) -> (w41:T8)  [unwired: 1 out]
  n77 = To Quad Integer(1:w32) -> (0:w33:i64)
  n78 = while {
    shift-left: w32 -> [w144]
    shift-right: [w143] -> _
    shift-left: w33 -> [w148]
    shift-right: [w149] -> _
    shift-left: w41 -> [w154]
    shift-right: [w155] -> _
    shift-left: w3 -> [w125]
    shift-right: [w156] -> _
    shift-left: w35 -> [w146]
    shift-right: [w157] -> _
    shift-left: w34 -> [w159]
    shift-right: [w158] -> _
    shift-left: w45 -> [w161]
    shift-right: [w160] -> _
    shift-left: w44 -> [w163]
    shift-right: [w162] -> _
    shift-right: [w140] -> _
    shift-left: w30 -> [w122]
    shift-right: [w135] -> _
    shift-left: w30 -> [w119]
    shift-right: [w133] -> _
    shift-left: w40 -> [w134]
    shift-right: [w132] -> _
    shift-left: w30 -> [w117]
    shift-right: [w127] -> _
    shift-left: w36 -> [w128]
    shift-right: [w115] -> _
    shift-left: w31 -> [w114]
    shift-right: [w113] -> _
    shift-left: w30 -> [w106]
    stop <- w147 stop-if-true
    w126 = 3  # Bytes per Word
    # "Sart with Save"
    # "Config Change"
    # "Current File in Byte"
    # "Header Lenght in Byte"
    # "Label Cluster"
    # "State machine with 6 states"
    # "Program runs continuously until\nEdit button is pressed in state 0"
    n79 = Unbundle By Name(w125) -> ("Speed Mode"=w105:i8, "Mon Channels"=w112:i32, "Bip Channels"=w111:i32, "Save Subset"=w110:i8, "Add Touchproofs"=w109:bool, "Add Sensors"=w108:bool, "Add Jazz"=w107:bool, "Add Anas"=w118:bool, "ADC Rate"=w121:i32, "Decimate Ratio"=w120:i32, "Save Box"=w116:u32)
    n80 = Wait (ms)(milliseconds to wait=u32 0) -> ()  [unwired: 1 out]
    n81 = Add(x="Buffer", y=i8 23) -> (x+y=w152:i8)
    n82 = Bundle("Speed Mode"=w105, "Save Subset"=w110, "Initially Channel Selection"=w122, "Add Touchproofs"=w109, "Mon Channels"=w112, "Bip Channels"=w111, "Add Sensors"=w108, "Initially Channel Selection"=w119, "Add Jazz"=w107, "Initially Channel Selection"=w106, "Add Anas"=w118, "Initially Channel Selection"=w117, "Save Box"=w116) -> (w123:T17)  [unwired: 1 out]
    n83 = call "SaveSelectDaisy.vi"("Save Selection Cluster"=w123) -> ("Number of Save Channels"=w124:i32)  [unwired: 1 out]
    n84 = Quotient & Remainder(x=w121, y=w120) -> (floor(x/y)=w139:i32)  [unwired: 1 out]
    n85 = Scale By Power Of 2(n="ScreenLength", x=1 ("X Scale.Range:Maximum")) -> (x*2^n=w129:i32)
    n86 = Scale By Power Of 2(n=w152, x=i64 1) -> (x*2^n=w150:i64)
    n87 = Scale By Power Of 2(n="Buffer", x=1) -> (x*2^n=w136:i32)
    n88 = Compound Arithmetic op=MULTIPLY(w126, w124, w139) -> (w141:i32)
    n89 = To Double Precision Float(number=w139) -> (double precision float=w145:dbl)
    n90 = case shown="4" w163 {
      tunnel: [w245 w1670 w2293 w2430 w2704 w5073] -> w162
      tunnel: w150 -> [_ w1454 _ _ w2543 _]
      tunnel: w145 -> [_ _ w2277 _ w2631 _]
      tunnel: w161 -> [w244 w1651 w2262 _ w2563 w5067]
      tunnel: [w244 w1651 w2262 w2421 w2562 w5046] -> w160
      tunnel: w159 -> [w243 w1667 w2309 _ w2700 w5071]
      tunnel: [w243 w1667 w2309 w2382 w2698 w5070] -> w158
      tunnel: [w242 w1458 w2264 w2427 w2613 w5057] -> w157
      tunnel: w141 -> [_ _ _ _ w2576 w5060]
      tunnel: [w236 w1441 w2267 w2415 w2686 w5045] -> w156
      tunnel: w125 -> [w186 w1503 w2267 w2414 w2618 w5045]
      tunnel: [w237 w1629 w2304 w2440 w2683 w5075] -> w155
      tunnel: w154 -> [w238 w1633 w2304 w2440 w2683 w5075]
      tunnel: [w241 w1668 w2308 w2384 w2702 w5044] -> w149
      tunnel: w148 -> [w241 w1668 w2308 _ w2697 w5072]
      tunnel: [w240 w1665 w2307 w2441 w2699 w5074] -> w147
      tunnel: w146 -> [w242 w1459 w2297 _ w2701 w5069]
      tunnel: w136 -> [_ _ w2300 _ _ _]
      tunnel: w144 -> [w239 w1669 w2306 _ w2696 w5068]
      tunnel: [w239 w1669 w2306 w2407 w2695 w5061] -> w143
      tunnel: w139 -> [_ _ _ _ w2637 _]
      tunnel: w122 -> [w202 w1666 w2305 w2402 w2688 w5066]
      tunnel: [w202 w1666 w2305 w2402 w2687 w5066] -> w140
      tunnel: w119 -> [w201 w1656 w2299 w2395 w2680 w5063]
      tunnel: [w201 w1656 w2299 w2395 w2679 w5063] -> w135
      tunnel: w134 -> [w222 w1655 w2280 w2425 w2678 w5065]
      tunnel: [w221 w1654 w2280 w2425 w2678 w5065] -> w133
      tunnel: w117 -> [w200 w1626 w2279 w2394 w2677 w5064]
      tunnel: [w200 w1626 w2279 w2394 w2676 w5064] -> w132
      tunnel: w129 -> [_ _ w2271 _ w2641 _]
      tunnel: w128 -> [w211 w1460 w2275 w2417 w2638 w5062]
      tunnel: [w210 w1460 w2275 w2417 w2640 w5062] -> w127
      tunnel: [w184 w1510 w2265 w2383 w2573 w5056] -> w115
      tunnel: w114 -> [_ w1510 w2265 w2383 w2572 w5056]
      tunnel: w106 -> [w169 w1482 w2263 w2375 w2570 w5047]
      tunnel: [w169 w1482 w2263 w2375 w2568 w5047] -> w113
      frame 0, Default {
        n91 = Unbundle By Name(w186) -> ("Save Subset"=w226:i8, "Add Touchproofs"=w231:bool, "Add Sensors"=w230:bool, "Add Jazz"=w216:bool, "Add Anas"=w177:bool, "Save Box"=w180:u32, "PauseOff"=w191:i32, "PauseOn"=w181:i32, "Save Path"=w182:path)
        n92 = Unbundle By Name(w211) -> ("Warning"=w215:i8, "Motherboard"=w214:i8, "ElecGain"=w213:i8, "RespSwitch"=w206:i8, "LineWidth"=w197:u8, "Cursor"=w199:u16, "PopupKiller"=w167:i8, "BreathBelt"=w164:i8)
        n93 = Boolean To (0,1)(Boolean=w216) -> (0, 1=w218:i16)
        n94 = Boolean To (0,1)(Boolean=w230) -> (0, 1=w229:i16)
        n95 = Boolean To (0,1)(Boolean=w177) -> (0, 1=w178:i16)
        n96 = Boolean To (0,1)(Boolean=w231) -> (0, 1=w228:i16)
        n97 = To Byte Integer(number=w197) -> (8bit integer=w196:i8)
        n98 = To Byte Integer(number=w199) -> (8bit integer=w198:i8)
        n99 = To Long Integer(number=w180) -> (32bit integer=w179:i32)
        n100 = To Long Integer(number=w226) -> (32bit integer=w183:i32)
        n101 = To Long Integer(number=w228) -> (32bit integer=w225:i32)
        n102 = To Long Integer(number=w218) -> (32bit integer=w217:i32)
        n103 = To Long Integer(number=w229) -> (32bit integer=w224:i32)
        n104 = To Long Integer(number=w178) -> (32bit integer=w176:i32)
        n105 = Unbundle By Name(w186) -> ("ADC Rate"=w185:i32)
        n106 = Build Array(w215, w214, w213, w206, w196, w198, w167, w164) -> (w212:i8[])
        n107 = Build Array(w183, w225, w224, w217, w176, w179, w191, w181) -> (w227:i32[])
        n108 = while {
          tunnel: ["Edit"] -> w240
          tunnel: [w429] -> w245
          shift-right: [w414] -> w237
          shift-left: w238 -> [w415]
          shift-right: [w378] -> w204
          shift-left: w227 -> [w349]
          shift-right: [w412] -> w221
          shift-left: w222 -> [w413]
          shift-right: [w344] -> w203
          shift-left: w212 -> [w347]
          shift-right: [w372] -> w175
          shift-left: w182 -> [w348]
          tunnel: w185 -> [w278]
          tunnel: [w247] -> w184
          stop <- w248 stop-if-true
          w252 = T5."Enabled" ("Disabled")
          w253 = T5."Disabled and Grayed Out" ("Disabled")
          w302 = 9  # Max Jazz Chan
          w304 = 0.2035  # 5th order sinc
          w340 = T18 1 items=["no dialog", "OK message", "continue or stop message", "OK message + warnings", "continue/stop + warnings"] ("type of dialog (OK msg:1)")
          w381 = "%d" ("Format String")
          w395 = 32  # Max Ana Chan
          w397 = 8  # Max Aux Chan
          w398 = 8  # Max Bip Chan
          w399 = 256  # Max Mon Chan
          w392 = FALSE ("Stop")
          w429 = 1  # Go to State 1    Configure
          n109 = Quotient & Remainder(x=w278, y=2048) -> (floor(x/y)=w315:i32)  [unwired: 1 out]
          n110 = Decrement(x=w315) -> (x-1=w314:i32)
          n111 = To Byte Integer(number=w314) -> (8bit integer=w313:i8)
          n112 = Less Or Equal To 0?(x=w278) -> (x <= 0?=w307:bool)
          n113 = Subtract(x="Decimation", y=w313) -> (x-y=w309:i8)
          n114 = local read "ScreenLength"() -> (w311:i32)
          n115 = Decrement(x=w309) -> (x-1=w279:i8)
          n116 = Scale By Power Of 2(n="Decimation", x=1) -> (x*2^n=w387:i32)
          n117 = Less Or Equal To 0?(x=w279) -> (x <= 0?=w308:bool)
          n118 = Or(x=w308, y=w307) -> (x .or. y?=w306:bool)
          n119 = Quotient & Remainder(x=w278, y=w387) -> (floor(x/y)=w416:i32)  [unwired: 1 out]
          n120 = case shown="False" w306 {
            tunnel: [w435 i32[] [] ("Disabled Items []")] -> w312
            tunnel: [w436 w440] -> w310
            tunnel: w311 -> [w437 w440]
            tunnel: w279 -> [w434 _]
            frame False {
              n121 = To Long Integer(number=w434) -> (32bit integer=w433:i32)
              n122 = Greater?(x=w433, y=w437) -> (0:w438:bool)
              n123 = for {
                N: w433 -> [_]
                tunnel: [w439] -> w435 mode=indexing
                i -> [w439]
              }
              n124 = Select(t=w433, s=w438, f=w437) -> (s? t:f=w436:i32)
            }
            frame True {
            }
          }
          n125 = Build Array("ScreenLength" ("key"), "FileLimit" ("key"), "FileAppend" ("key"), "RecTimeLimit" ("key"), "Decimation" ("key"), "Buffer" ("key"), "MonScale" ("key"), "MonLP" ("key"), "MonLPfreq" ("key"), "MonHP" ("key"), "MonHPfreq" ("key"), "Channels" ("key"), "AddTP" ("key"), "Reference" ("key"), "TrigCode" ("key"), "BipScale" ("key"), "BipLP" ("key"), "BipLPfreq" ("key"), "BipHP" ("key"), "BipHPfreq" ("key"), "Offset" ("key"), "OffsetScale" ("key"), "AvgTrigLog" ("key"), "AvgSweep" ("key"), "AvgLP" ("key"), "AvgLPfreq" ("key"), "AvgHP" ("key"), "AvgHPfreq" ("key"), "AvgAutoscale" ("key"), "AvgScale" ("key"), "AvgAbsReject" ("key"), "AvgRelReject" ("key"), "GsrScale" ("key"), "ErgoScale" ("key"), "ErgoLP" ("key"), "RespScale" ("key"), "PletScale" ("key"), "TempScale" ("key"), "AuxReset" ("key"), "JazzOn" ("key"), "JazzReset" ("key"), "AnaScale" ("key"), "AnaLP" ("key"), "AnaLPfreq" ("key"), "AnaHP" ("key"), "AnaHPfreq" ("key"), "AnaReset" ("key"), "AnaOffset" ("key")) -> (w318:string[])
          n126 = To Double Precision Float(number=w416) -> (double precision float=w246:dbl)
          "Sample Rate" <- w246
          n127 = Multiply(x=w246, y=w304) -> (x*y=→"Bandwidth (3dB)":dbl)
          n128 = call "AVTCP-Sample Rate FGV.vi"("Value in"=w246) -> ()  [unwired: 6 in, 1 out]
          n129 = property class="App"() -> ("Application:Kind"=w326:T3)  [unwired: 2 in, 2 out]
          "Application:Kind" <- w326
          n130 = First Call?() -> (First Call?: T/F=w373:bool)
          n131 = Build Array("LocalPort" ("key"), "TCPsubset" ("key"), "TCPaddTP" ("key"), "TCPaddSens" ("key"), "TCPaddJazz" ("key"), "TCPaddAnas" ("key"), "TCPaddTrig" ("key")) -> (w334:string[])
          n132 = Or(x="Load Configuration File", y=w373) -> (x .or. y?=w408:bool)
          n133 = Build Array("MonFree" ("key"), "RefFree" ("key"), "BipFree" ("key"), "AvgTrigSel" ("key"), "MonFreeAvg1" ("key"), "RefFreeAvg1" ("key"), "MonFreeAvg2" ("key"), "RefFreeAvg2" ("key"), "AuxFree" ("key"), "JazzFree" ("key"), "AnaFree" ("key")) -> (w368:string[])
          n134 = local write "ScreenLength"(w310) -> ()
          n135 = property on="ScreenLength" class="Ring (strict)"("Disabled Items []"=w312) -> ()  [unwired: 2 in, 2 out]
          n136 = Equal?(x=w326, y=T3."Run Time System") -> (x = y?=w325:bool)
          n137 = Build Array("Warning" ("key"), "Motherboard" ("key"), "ElecGain" ("key"), "RespSwitch" ("key"), "LineWidth" ("key"), "Cursor" ("key"), "PopupKiller" ("key"), "BreathBelt" ("key")) -> (w317:string[])
          n138 = Select(t=i8 1, s=w408, f=i8 0 ("t")) -> (s? t:f=w410:i8)
          n139 = Build Array("Subset" ("key"), "Touchproofs" ("key"), "Sensors" ("key"), "Jazz" ("key"), "Anas" ("key"), "SaveBox" ("key"), "PauseOff" ("key"), "PauseOn" ("key"), "SavePath" ("key")) -> (w390:string[])
          n140 = Select(t=i8 2, s="Save Configuration File", f=w410) -> (s? t:f=w411:i8)
          n141 = case shown="0, Default" w411 {
            tunnel: w415 -> [w446 w492 w1100]
            tunnel: w373 -> [_ w451 _]
            tunnel: [w446 w491 w1100] -> w414
            tunnel: [w445 w490 w1097] -> w378
            tunnel: w349 -> [w445 w489 w1097]
            tunnel: w413 -> [w444 w487 w1113]
            tunnel: [w444 w488 w1113] -> w412
            tunnel: w318 -> [_ w486 w1106]
            tunnel: "Labels" -> [_ w485 w1104]
            tunnel: "Selectors" ("section") -> [_ w484 w1105]
            tunnel: "FreeChoice" ("section") -> [_ w483 w1099]
            tunnel: "Save" ("section") -> [_ w482 w1098]
            tunnel: w399 -> [_ w481 w1103]
            tunnel: w398 -> [_ w480 w1102]
            tunnel: w397 -> [_ w479 w1101]
            tunnel: w395 -> [_ w478 w1084]
            tunnel: w390 -> [_ w477 w1096]
            tunnel: "System" -> [_ w476 w1094]
            tunnel: [w443 w475 w1095] -> w344
            tunnel: w347 -> [w443 w473 w1095]
            tunnel: w317 -> [_ w474 w1093]
            tunnel: w348 -> [w442 w472 w1092]
            tunnel: w334 -> [_ w471 w1091]
            tunnel: [w442 w470 w1092] -> w372
            tunnel: w368 -> [_ w469 w1090]
            tunnel: "TCP" ("section") -> [_ w452 w1089]
            tunnel: w325 -> [_ w450 w1088]
            tunnel: "*.cfg" ("pattern") -> [_ w449 w1086]
            tunnel: "Configuring File" ("pattern label") -> [_ w448 w1085]
            tunnel: w302 -> [_ w447 w1083]
            frame 0, Default {
            }
            frame 1 {
              w462 = "Default.cfg"  # Default Configuration File
              # "Does File Exist?"
              n142 = Current VI's Path() -> (path=w497:path)
              n143 = property class="App"() -> (reference out=w468:refnum<vi>, "Application:Command Line Arguments"=w467:string[])  [unwired: 2 in, 1 out]
              n144 = Strip Path(path=w497) -> (stripped path=w496:path)  [unwired: 1 out]
              n145 = case shown="True" w450 {
                tunnel: w496 -> [w1080 w1082]
                tunnel: [w1080 w1081] -> w460
                frame False {
                }
                frame True {
                  n146 = Strip Path(path=w1082) -> (stripped path=w1081:path)  [unwired: 1 out]
                }
              }
              n147 = Index Array(array=w467, index=1) -> (element=w463:string)
              n148 = Close Reference(reference=w468) -> (error out=w461:errorcluster)  [unwired: 1 in]
              n149 = Not Equal?(x=w463, y="") -> (x != y?=w464:bool)
              n150 = Select(t=w463, s=w464, f=w462) -> (s? t:f=w457:string)
              n151 = Build Path(base path=w460, name or relative path=w457) -> (appended path=w498:path)
              n152 = File/Directory Info(path=w498, error in=w461) -> (path out=w459:path, error out=w456:errorcluster)  [unwired: 5 out]
              n153 = Unbundle By Name(w456) -> ("code"=w495:i32)
              n154 = Not Equal?(x=w495, y=7 ("code")) -> (x != y?=w493:bool)
              n155 = And(x=w493, y=w451) -> (x .and. y?=w458:bool)
              n156 = case shown="False" w458 {
                tunnel: w460 -> [w505 _]
                tunnel: [w504 w509] -> w454
                tunnel: w459 -> [_ w509]
                tunnel: w457 -> [w502 _]
                tunnel: [w503 w508] -> w453
                tunnel: w456 -> [_ w507]
                tunnel: [w501 w507] -> w455
                tunnel: w449 -> [w500 _]
                tunnel: w448 -> [w499 _]
                frame False {
                  n157 = File Dialog(4:w499, 6:w500, 7:"Enter filename:" ("prompt"), 9:w502, 11:w505) -> (0:w501:errorcluster, 1:w503:bool, 3:w504:path)  [unwired: 1 in, 2 out]
                }
                frame True {
                  w508 = FALSE  # Cancelled?
                }
              }
              n158 = case shown="False" w453 {
                tunnel: w492 -> [w553 w1079]
                tunnel: [w547 w1079] -> w491
                tunnel: w454 -> [w513 _]
                tunnel: [w548 w1078] -> w490
                tunnel: w489 -> [_ w1078]
                tunnel: [w549 w1077] -> w488
                tunnel: w487 -> [_ w1077]
                tunnel: w486 -> [w539 _]
                tunnel: w485 -> [w538 _]
                tunnel: w484 -> [w537 _]
                tunnel: w483 -> [w536 _]
                tunnel: w482 -> [w535 _]
                tunnel: w481 -> [w534 _]
                tunnel: w480 -> [w533 _]
                tunnel: w479 -> [w532 _]
                tunnel: w478 -> [w531 _]
                tunnel: w477 -> [w528 _]
                tunnel: w476 -> [w527 _]
                tunnel: [w526 w1076] -> w475
                tunnel: w474 -> [w525 _]
                tunnel: w473 -> [_ w1076]
                tunnel: w472 -> [_ w1075]
                tunnel: w471 -> [w522 _]
                tunnel: [w521 w1075] -> w470
                tunnel: w469 -> [w520 _]
                tunnel: w455 -> [w512 _]
                tunnel: w452 -> [w518 _]
                tunnel: w447 -> [w514 _]
                frame False {
                  w523 = T18 1 items=["no dialog", "OK message", "continue or stop message", "OK message + warnings", "continue/stop + warnings"] ("type of dialog (OK msg:1)")
                  w549 = TRUE  # Config Changed
                  n159 = Path To String(path=w513) -> (string=→"Current Filepath":string)
                  n160 = call <vilib>:"Open Config Data.vi"("error in (no error)"=w512, "configuration file path"=w513) -> ("error out"=w511:errorcluster, "refnum"=w510:T19)  [unwired: 7 in, 1 out]
                  n161 = stacked-sequence {
                    seq-local: [_ w644 _ _ _ _] -> [_ _ w837 _ _ _]
                    seq-local: [_ w643 _ _ _ _] -> [_ _ w836 _ _ _]
                    seq-local: [_ _ w835 _ _ _] -> [_ _ _ w968 _ _]
                    seq-local: [_ _ w834 _ _ _] -> [_ _ _ w967 _ _]
                    seq-local: [_ _ _ w965 _ _] -> [_ _ _ _ w1024 _]
                    seq-local: [_ _ _ w964 _ _] -> [_ _ _ _ w1023 _]
                    seq-local: [w562 _ _ _ _ _] -> [_ w646 _ _ _ _]
                    seq-local: [w563 _ _ _ _ _] -> [_ w647 _ _ _ _]
                    seq-local: [_ _ _ _ w1002 _] -> [_ _ _ _ _ w1046]
                    seq-local: [_ _ _ _ w1001 _] -> [_ _ _ _ _ w1045]
                    seq-local: [w556 _ _ _ _ _] -> [_ w649 _ _ _ _]
                    seq-local: [w554 _ _ _ _ _] -> [_ _ w828 _ _ _]
                    tunnel: w553 -> [_ w672 _ _ _ _]
                    tunnel: w510 -> [w567 _ _ _ _ _]
                    tunnel: w511 -> [w566 _ _ _ _ _]
                    tunnel: [_ _ _ _ _ w1042] -> w550
                    tunnel: [_ _ _ _ _ w1041] -> w545
                    tunnel: [_ _ _ _ w1022 _] -> w548
                    tunnel: [_ w658 _ _ _ _] -> w547
                    tunnel: [_ w654 _ _ _ _] -> w517
                    tunnel: [_ _ w831 _ _ _] -> w515
                    tunnel: [_ _ _ w963 _ _] -> w530
                    tunnel: [_ _ _ _ w1015 _] -> w540
                    tunnel: w539 -> [_ _ w830 _ _ _]
                    tunnel: w538 -> [_ w648 _ _ _ _]
                    tunnel: w537 -> [_ _ w829 _ _ _]
                    tunnel: w536 -> [_ _ _ w966 _ _]
                    tunnel: w535 -> [_ _ _ _ w1018 _]
                    tunnel: w534 -> [_ w642 _ _ _ _]
                    tunnel: w533 -> [_ w652 _ _ _ _]
                    tunnel: w532 -> [_ w657 _ _ _ _]
                    tunnel: w531 -> [_ w650 _ _ _ _]
                    tunnel: w528 -> [_ _ _ _ w1004 _]
                    tunnel: w527 -> [w564 _ _ _ _ _]
                    tunnel: [w568 _ _ _ _ _] -> w516
                    tunnel: [w557 _ _ _ _ _] -> w526
                    tunnel: w525 -> [w565 _ _ _ _ _]
                    tunnel: w513 -> [w560 _ _ _ _ _]
                    tunnel: w522 -> [_ _ _ _ _ w1044]
                    tunnel: [_ _ _ _ w1010 _] -> w521
                    tunnel: w520 -> [_ _ _ w969 _ _]
                    tunnel: [_ _ _ _ _ w1038] -> w519
                    tunnel: w518 -> [_ _ _ _ _ w1043]
                    tunnel: w514 -> [_ w636 _ _ _ _]
                    frame #0 {
                      # "ElecGain"
                      # "LineWidth"
                      # "Not Found"
                      n162 = for {
                        shift-right: [w575] -> w563
                        shift-left: w567 -> [w589]
                        shift-right: [w572] -> w562
                        shift-left: w566 -> [w588]
                        tunnel: [w571] -> w557 mode=indexing
                        tunnel: [w582] -> w561 mode=indexing
                        tunnel: w564 -> [w578]
                        tunnel: w565 -> [w573] mode=indexing
                        tunnel: w560 -> [w574]
